vi "PS4AxisNormalize (SubVI).vi"(6 "NormalizeTo":dbl=450.0, 10 "PS4 Thumbstick":cluster{"Array":i32[], "Array":i32[]}) -> (1 "Y":dbl, 2 "X":dbl)   [LabVIEW 2020]
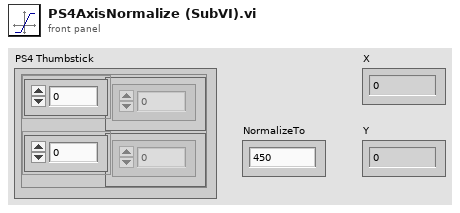
[diagram p1: front panel]
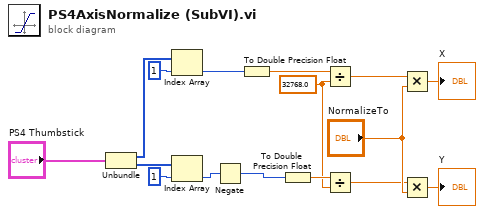
[diagram p0: block diagram]
diagram:
  w6 = 32768.0 ("y")
  n1 = Unbundle("PS4 Thumbstick") -> ("Array"=w11:i32[], "Array"=w12:i32[])
  n2 = Index Array(array=w11, index=1) -> (element=w8:i32)
  n3 = Index Array(array=w12, index=1) -> (element=w15:i32)
  n4 = Negate(x=w15) -> (-x=w10:i32)
  n5 = To Double Precision Float(number=w8) -> (double precision float=w7:dbl)
  n6 = To Double Precision Float(number=w10) -> (double precision float=w9:dbl)
  n7 = Divide(x=w7, y=w6) -> (x/y=w2:dbl)
  n8 = Divide(x=w9, y=w6) -> (x/y=w1:dbl)
  n9 = Multiply(x=w2, y="NormalizeTo") -> (x*y=→"X":dbl)
  n10 = Multiply(x=w1, y="NormalizeTo") -> (x*y=→"Y":dbl)
